vi "Create.vi"(8 "error in (no error)":errorcluster, 10 "Dependencies":T1[](array[typedef]), 11 "Package Info":T2) -> (0 "error out":errorcluster, 3 "GPack File out":refnum<class "GPack File.lvclass">)   [LabVIEW 2020, in "GPack.lvlib" / "GPack File.lvclass"]
uses:
  GPack File.lvclass
  Package Info.ctl
  Dependency.ctl
  GPack File.lvclass/GPack File.ctl
  GPack.lvlib
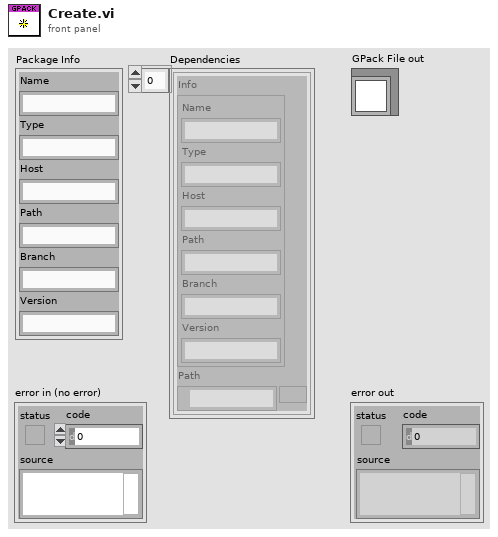
[diagram p1: front panel]
types:
  T1 = typedef "GPack.lvlib/Dependency.ctl" = cluster{"Info":T2, "Path":path}
  T2 = typedef "GPack.lvlib/Package Info.ctl" = cluster{"Name":string, "Type":string, "Host":string, "Path":string, "Branch":string, "Version":string}
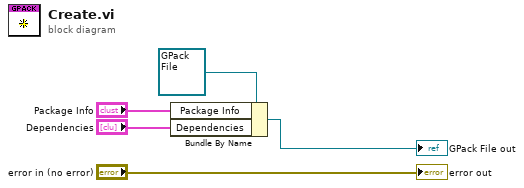
[diagram p0: block diagram]
diagram:
  n1 = Bundle By Name(cluster=refnum<class "GPack File.lvclass"> refnum ("GPack File in"), "Package Info"="Package Info", "Dependencies"="Dependencies") -> (→"GPack File out":refnum<class "GPack File.lvclass">)
  "error out" <- "error in (no error)"
